vi "Test Locally.vi"   [LabVIEW 2023]
uses:
  Host Reply Time Test Actor/Host Reply Time Test Actor/Host Reply Time Test Actor.lvclass
  C:/Program Files/National Instruments/LabVIEW 2023/vi.lib/ActorFramework/Actor/Actor.lvclass
  Target Reply Time Test Actor/Target Reply Time Test Actor/Target Reply Time Test Actor.lvclass
  Host Reply Time Test Actor/Host Reply Time Test Actor/Host Reply Time Test Actor.lvclass/Host Reply Time Test Actor.ctl
  Target Reply Time Test Actor/Target Reply Time Test Actor/Target Reply Time Test Actor.lvclass/Target Reply Time Test Actor.ctl
  <vilib>/ni/Actors/Network Endpoint Actors/Protocols/Network Stream Strategy/Netowrk Stream Listener/Network Stream Listener.lvclass
  C:/Program Files/National Instruments/LabVIEW 2023/vi.lib/ni/Actors/Network Endpoint Actors/Abstract Classes/Message Stream/Message Stream.lvclass
  <vilib>/ni/Actors/Network Endpoint Actors/Protocols/Network Stream Strategy/Network Stream Initiator/Network Stream Initiator.lvclass
  <vilib>/ActorFramework/Actor/Actor.lvclass
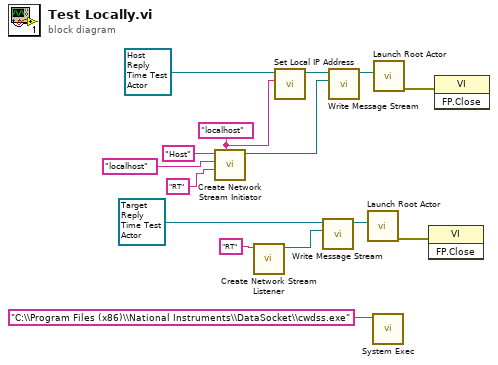
[diagram p0: block diagram]
diagram:
  w2 = "localhost" ("Local Address")
  n1 = call <vilib>:"Create Network Stream Initiator.vi"("Local Address"=w2, "Remote Name"="RT", "Remote Address"="localhost", "Name"="Host") -> ("Network Stream Initiator out"=w10:refnum<class "Network Stream Initiator.lvclass">)  [unwired: 7 in]
  n2 = call <vilib>:"Create Network Stream Listener.vi"("Name"="RT" ("Remote Name")) -> ("Network Stream Listener"=w7:refnum<class "Network Stream Listener.lvclass">)  [unwired: 10 in]
  n3 = call "Set Local IP Address.vi"("Local IP Address"=w2, "Host Reply Time Test Actor in"=refnum<class "Host Reply Time Test Actor.lvclass"> refnum ("Host Reply Time Test Actor.lvlib:Host Reply Time Test Actor.lvclass")) -> ("Host Reply Time Test Actor out"=w3:refnum<class "Host Reply Time Test Actor.lvclass">)  [unwired: 9 in]
  n4 = call "Write Message Stream.vi"("Message Stream.lvclass"=w7, "Target Reply Time Test Actor in"=refnum<class "Target Reply Time Test Actor.lvclass"> refnum ("Target Reply Time Test Actor.lvlib:Target Reply Time Test Actor.lvclass")) -> ("Target Reply Time Test Actor out"=w8:refnum<class "Target Reply Time Test Actor.lvclass">)  [unwired: 9 in]
  n5 = call "Write Message Stream.vi"("Message Stream.lvclass"=w10, "Host Reply Time Test Actor in"=w3) -> ("Host Reply Time Test Actor out"=w11:refnum<class "Host Reply Time Test Actor.lvclass">)  [unwired: 8 in, 1 out]
  n6 = call <vilib>:"Launch Root Actor.vi"("Actor"=w8) -> ("error out"=w9:errorcluster)  [unwired: 9 in, 1 out]
  n7 = call <vilib>:"System Exec.vi"("command line"="C:\\Program Files (x86)\\National Instruments\\DataSocket\\cwdss.exe") -> ()  [unwired: 7 in, 4 out]
  n8 = call <vilib>:"Launch Root Actor.vi"("Actor"=w11) -> ("error out"=w15:errorcluster)  [unwired: 9 in, 1 out]
  n9 = invoke class="VI" method="FP.Close"(error in=w9) -> ()  [unwired: 2 in, 3 out]
  n10 = invoke class="VI" method="FP.Close"(error in=w15) -> ()  [unwired: 2 in, 3 out]
